vi "encode error estimates.vi"(10 "state":T1) -> (2 "pos and vel":u32)   [LabVIEW 2010]
uses:
  FPGA tracking/integrating single axis kalman state.ctl
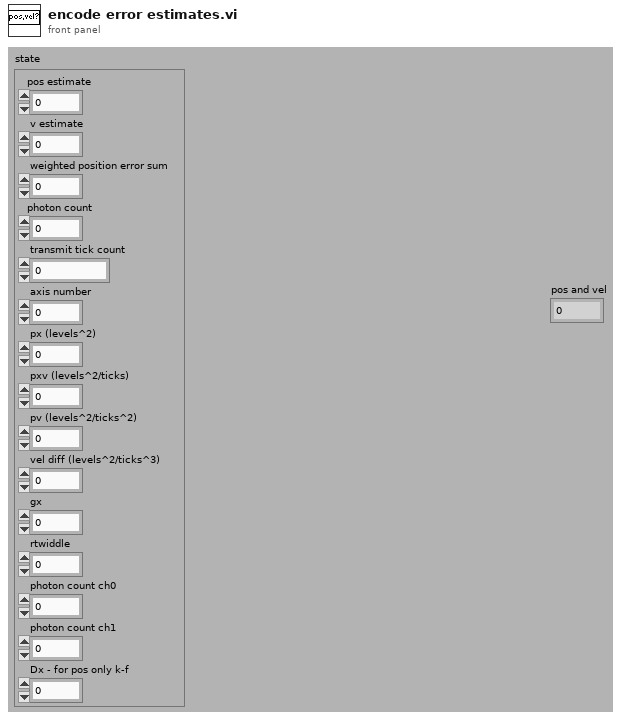
[diagram p1: front panel]
types:
  T1 = typedef "integrating single axis kalman state.ctl" = cluster{"pos estimate":fxp<+/-,32,16>, "v estimate":fxp<+/-,16,0>, "weighted position error sum":fxp<+/-,32,32>, "photon count":u32, "transmit tick count":u32, "axis number":u8, "px (levels^2)":fxp<+,32,19>, "pxv (levels^2/ticks)":fxp<+,32,2>, "pv (levels^2/ticks^2)":fxp<+,32,-14>, "vel diff (levels^2/ticks^3)":fxp<+,24,-22>, "gx":fxp<+,16,8>, "rtwiddle":fxp<+,16,26>, "photon count ch0":u32, "photon count ch1":u32, "Dx - for pos only k-f":fxp<+,32,19>}
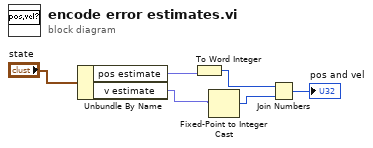
[diagram p0: block diagram]
diagram:
  n1 = Unbundle By Name("state") -> ("pos estimate"=w5:fxp<+/-,32,16>, "v estimate"=w2:fxp<+/-,16,0>)
  n2 = To Word Integer(number=w5) -> (16bit integer=w4:i16)
  n3 = Fixed-Point to Integer Cast(1:w2) -> (0:w1:i16)
  n4 = Join Numbers(hi=w4, lo=w1) -> ((hi.lo)=→"pos and vel":u32)
